vi "_API_BINANCE_GET_USDT_FUTURES_lastTradeOnSymbol.vi"(0 "BinanceAPI in":refnum<class "BinanceAPI_.lvclass">, 5 "CurrentAllOpenOrders":cluster{"symbol (eg. BTCUSDT)":string}, 11 "error in (no error)":errorcluster) -> (4 "BinanceAPI out":refnum<class "BinanceAPI_.lvclass">, 6 "data":T1, 14 "Body":string, 15 "error out":errorcluster)   [LabVIEW 2022 SP3, in "BinanceAPI_.lvclass"]
doc: "https://binance-docs.github.io/apidocs/futures/en/#account-trade-list-user_data"
uses:
  BinanceAPI_.lvclass
  BinanceAPI_.lvclass/BinanceAPI_.ctl
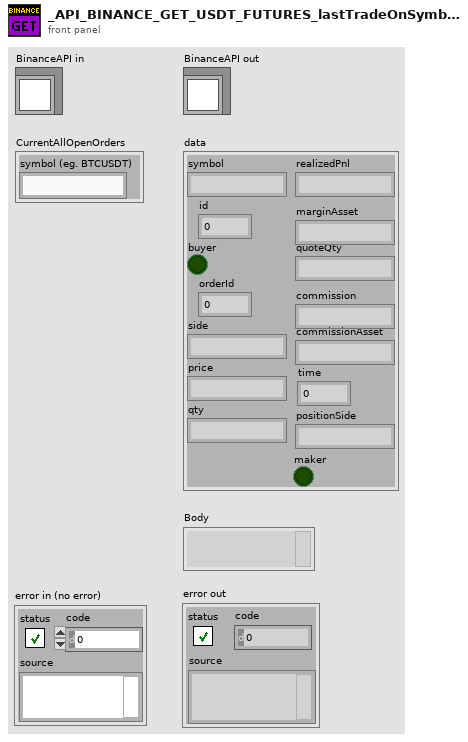
[diagram p1: front panel]
types:
  T1 = cluster{"symbol":string, "id":dbl, "buyer":bool, "orderId":dbl, "side":string, "price":string, "qty":string, "realizedPnl":string, "marginAsset":string, "quoteQty":string, "commission":string, "commissionAsset":string, "time":dbl, "positionSide":string, "maker":bool}
  T2 = cluster{"symbol":string, "id":dbl, "buyer":bool, "orderId":dbl, "side":string, "price":string, "qty":string, "realizedPnl":string, "marginAsset":string, "quoteQty":string, "commission":string, "commissionAsset":string, "time":dbl, "positionSide":string, "maker":bool}[]
  T3 = enum16{"SPOT", "USDT_FUTURES", "COIN_FUTURES", "VANILLA"}
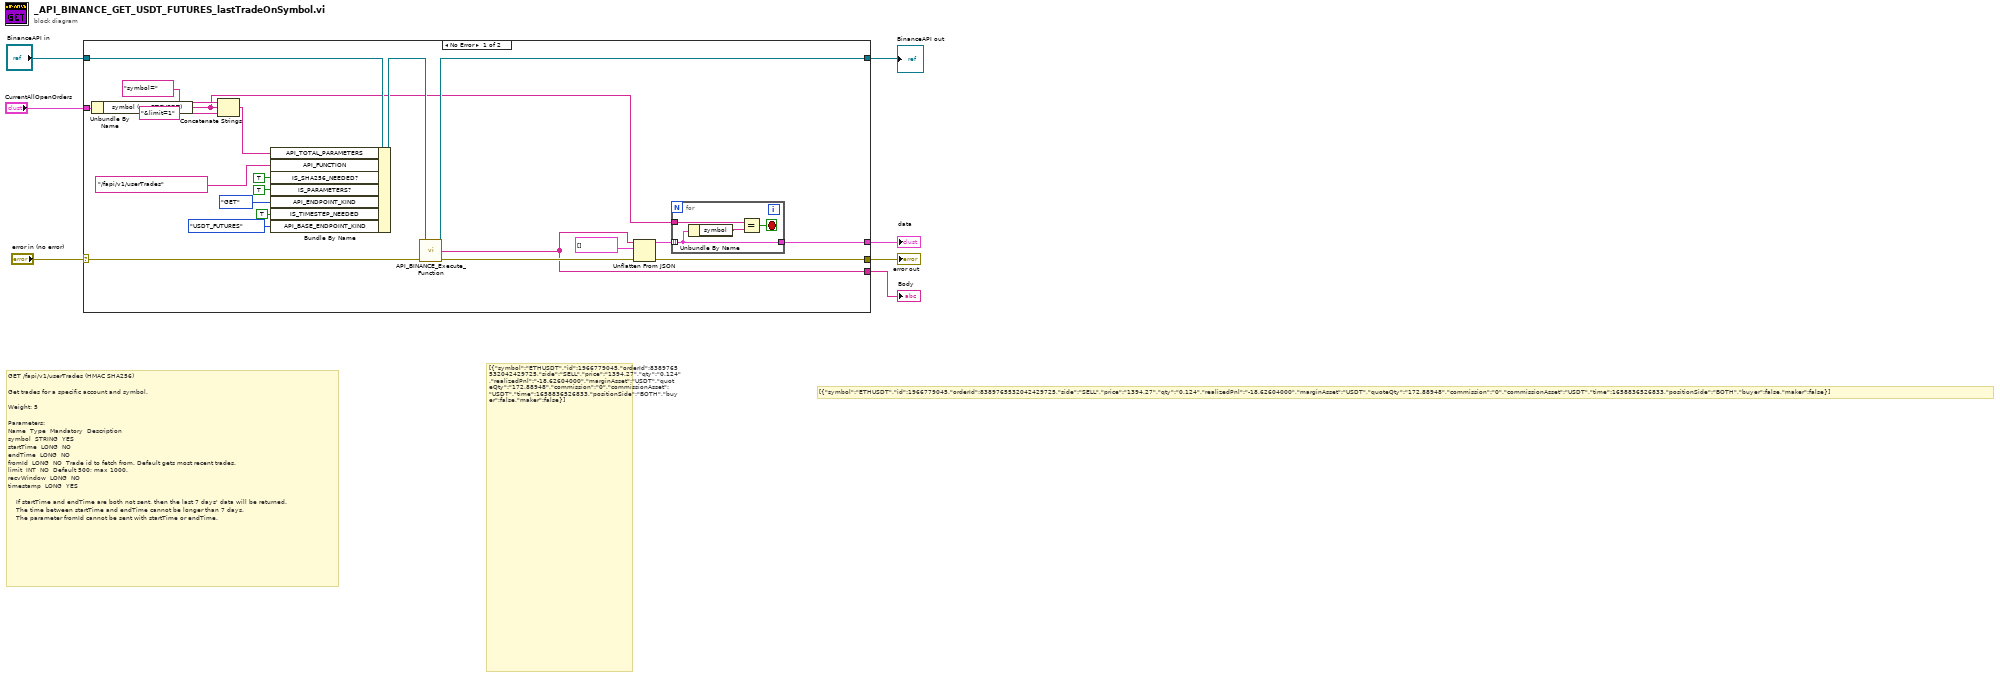
[diagram p0: block diagram]
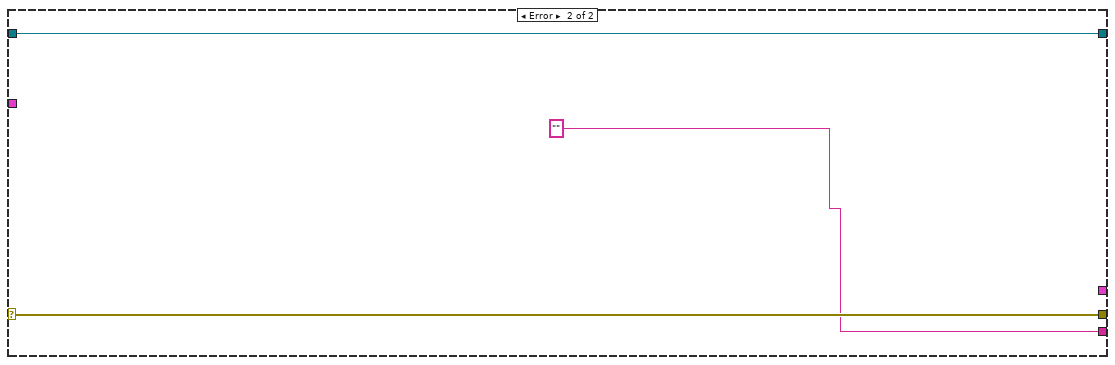
[diagram p2: hidden frame]
diagram:
  # "[{\"symbol\":\"ETHUSDT\",\"id\":1966779045,\"orderId\":8389765532042429725,\"side\":\"SELL\",\"price\":\"1394.27\",\"qty\":\"0.124\",\"realizedPnl\":\"-18.62604000\",\"marginAsset\":\"USDT\",\"quoteQty\":\"172.88948\",\"commission\":\"0\",\"commissionAsset\":\"USDT\",\"time\":1658836526833,\"positionSide\":\"BOTH\",\"buyer\":false,\"maker\":false}]"
  # "[{\"symbol\":\"ETHUSDT\",\"id\":1966779045,\"orderId\":8389765532042429725,\"side\":\"SELL\",\"price\":\"1394.27\",\"qty\":\"0.124\",\"realizedPnl\":\"-18.62604000\",\"marginAsset\":\"USDT\",\"quoteQty\":\"172.88948\",\"commission\":\"0\",\"commissionAsset\":\"USDT\",\"time\":1658836526833,\"positionSide\":\"BOTH\",\"buyer\":false,\"maker\":false}]"
  # "GET /fapi/v1/userTrades (HMAC SHA256)\n\nGet trades for a specific account and symbol.\n\nWeight: 5\n\nParameters:\nName \tType \tMandatory \tDescription\nsymbol \tSTRING \tYES \t\nstartTime \tLONG \tNO \t\nendTime \tLONG \tNO \t\nfromId \tLONG \tNO \tTrade id to fetch from. Default gets most recent trades.\nlimit \tINT \tNO \tDefault 500; max 1000.\nrecvWindow \tLONG \tNO \t\ntimestamp \tLONG \tYES \t\n\n    If startTime and endTime are both not sent, then the last 7 days' data will be returned.\n    The time between startTime and endTime cannot be longer than 7 days.\n    The parameter fromId cannot be sent with startTime or endTime."
  n1 = case shown="No Error" "error in (no error)" {
    selector: "error in (no error)" -> [w18 w35]
    tunnel: [w13 w35] -> w5
    tunnel: [w19 w34] -> w1
    tunnel: "BinanceAPI in" -> [w28 w34]
    tunnel: "CurrentAllOpenOrders" -> [w21 _]
    tunnel: [w12 "" ("Header")] -> w4
    tunnel: [w8 _] -> w3
    frame No Error {
      n2 = Unbundle By Name(w21) -> ("symbol (eg. BTCUSDT)"=w9:string)
      n3 = Concatenate Strings("symbol=", w9, "&limit=1" ("string")) -> (w22:string)
      n4 = Bundle By Name(cluster=w28, "API_TOTAL_PARAMETERS"=w22, "API_FUNCTION"="/fapi/v1/userTrades", "IS_SHA256_NEEDED?"=TRUE, "IS_PARAMETERS?"=TRUE, "API_ENDPOINT_KIND"=enum16{"POST", "DELETE", "GET", "PUT"}."GET", "IS_TIMESTEP_NEEDED"=TRUE, "API_BASE_ENDPOINT_KIND"=T3."USDT_FUTURES") -> (w20:refnum<class "BinanceAPI_.lvclass">)
      n5 = call "API_BINANCE_Execute_Function.vi"("BinanceAPI in"=w20, "error in (no error)"=w18) -> ("BinanceAPI out"=w19:refnum<class "BinanceAPI_.lvclass">, "Body"=w12:string, "error out"=w17:errorcluster)  [unwired: 9 in, 2 out]
      n6 = Unflatten From JSON(JSON string=w12, type and defaults=T2 [], error in (no error)=w17) -> (value=w10:T2, error out=w13:errorcluster)  [unwired: 4 in]
      n7 = for {
        tunnel: w10 -> [w29] mode=indexing
        tunnel: w9 -> [w31]
        tunnel: [w29] -> w8
        stop <- w30 stop-if-true
        n8 = Unbundle By Name(w29) -> ("symbol"=w32:string)
        n9 = Equal?(x=w31, y=w32) -> (x = y?=w30:bool)
      }
    }
    frame Error {
    }
  }
  "error out" <- w5
  "Body" <- w4
  "data" <- w3
  "BinanceAPI out" <- w1
